vi "Universal Obstacle Drive - Clark and David.vi"(11 "Accelerometer":dbl) -> (2 "Complete":bool, 3 "Arcade Drive":T1)   [LabVIEW 2015]
uses:
  Universal Drive Through - Clark and David.ctl
panel:
  in  "Count":dbl
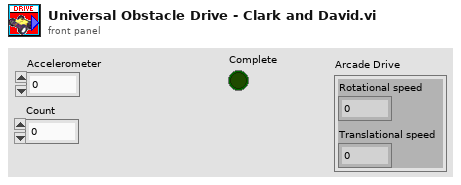
[diagram p1: front panel]
types:
  T1 = cluster{"Translational speed":dbl, "Rotational speed":dbl}
  T2 = typedef "Universal Drive Through - Clark and David.ctl" = enum16{"Ready", "Move", "Stop"}
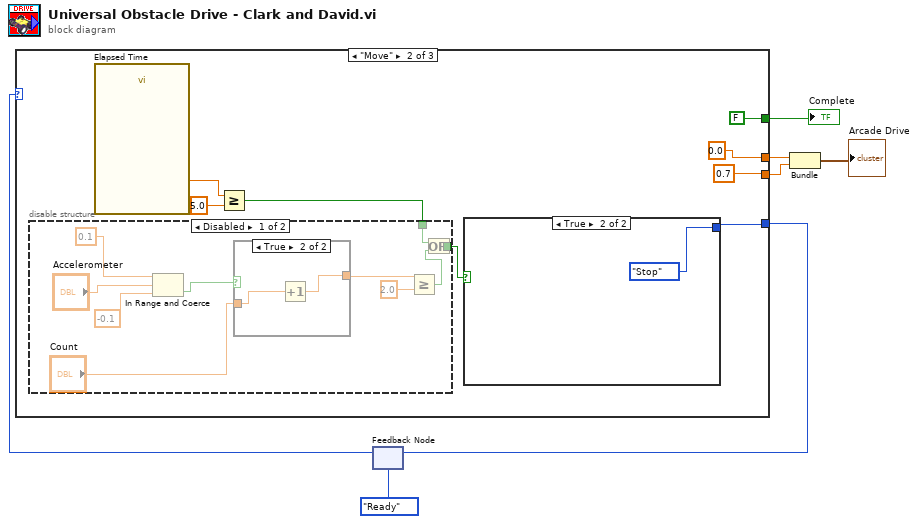
[diagram p0: block diagram]
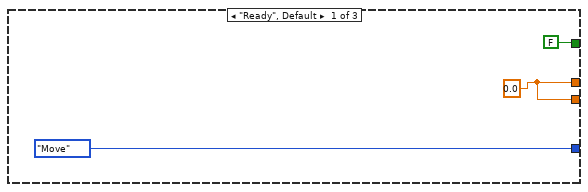
[diagram p2: hidden frame]
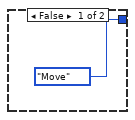
[diagram p5: hidden frame]
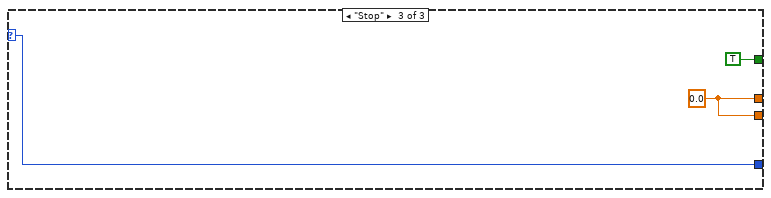
[diagram p6: hidden frame]
diagram:
  n1 = feedback #1(Universal_Drive_Through_-_Clark_and_David."Ready") -> (w6:T2)
  n2 = case shown="\"Move\"" w6 {
    selector: w6 -> [_ _ w36]
    tunnel: [Universal_Drive_Through_-_Clark_and_David."Move" w15 w36] -> w5
    tunnel: [FALSE FALSE TRUE] -> w4
    tunnel: [w8 0.0 w34] -> w3
    tunnel: [w8 0.7 w34] -> w2
    frame "Ready", Default {
      w8 = 0.0 ("Motor speed")
    }
    frame "Move" {
      n3 = call "Elapsed Time"() -> ("Elapsed Time (s)"=w18:dbl)  [unwired: 12 in, 7 out]
      n4 = Greater Or Equal?(x=w18, y=5.0) -> (x >= y?=w16:bool)
      n5 = disable-structure shown="Disabled" {
        disable-tunnel: w16 -> [w25 _]
        disable-tunnel: [w19 _] -> w13
        frame Disabled {
          n6 = In Range and Coerce(upper limit=0.1, x="Accelerometer", lower limit=-0.1) -> (In Range?=w24:bool)  [unwired: 1 out]
          n7 = case shown="True" w24 {
            tunnel: "Count" -> [w29 w31]
            tunnel: [w29 w30] -> w21
            frame False {
            }
            frame True {
              n8 = Increment(x=w31) -> (x+1=w30:dbl)
            }
          }
          n9 = Greater Or Equal?(x=w21, y=2.0) -> (x >= y?=w20:bool)
          n10 = Or(x=w25, y=w20) -> (x .or. y?=w19:bool)
        }
        frame Enabled {
        }
      }
      n11 = case shown="True" w13 {
        tunnel: [Universal_Drive_Through_-_Clark_and_David."Move" Universal_Drive_Through_-_Clark_and_David."Stop"] -> w15
        frame False {
        }
        frame True {
        }
      }
    }
    frame "Stop" {
      w34 = 0.0
    }
  }
  "Complete" <- w4
  n12 = feedback-in #1(w5) -> ()
  n13 = Bundle("Motor speed"=w3, "Motor speed"=w2) -> (→"Arcade Drive":cluster{"Motor speed":dbl, "Motor speed":dbl})  [unwired: 1 in]
